vi "tcp_monitor_read_a_frame.vi"(7 "Save":bool, 8 "error in (no error)":errorcluster, 11 "TCP Network Connection in":refnum<k5>) -> (0 "error out":errorcluster, 2 "DataString":string, 3 "TCP Network Connection out":refnum<k5>)   [LabVIEW 2022 SP3]
uses:
  Global 1.vi
panel:
  out "error out 2":errorcluster
  out "length string":string
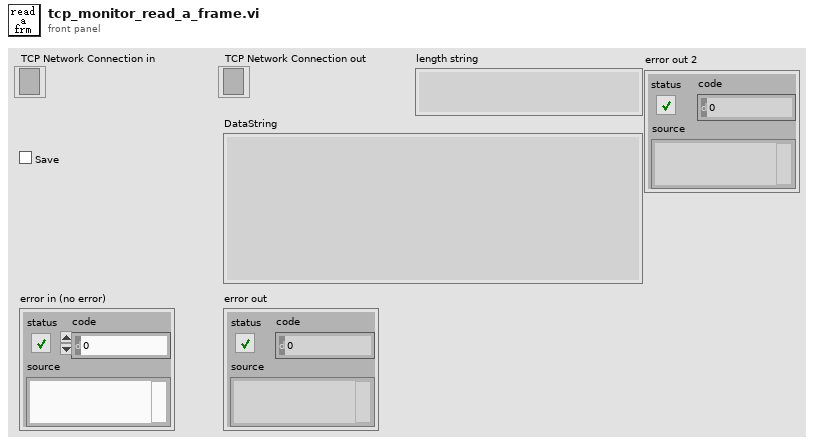
[diagram p1: front panel]
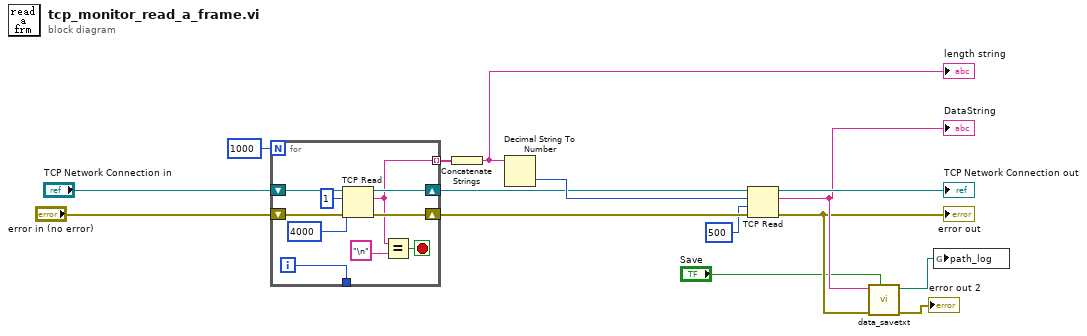
[diagram p0: block diagram]
diagram:
  n1 = for {
    N: 1000 -> [_]
    shift-right: [w24] -> w9
    shift-left: "TCP Network Connection in" -> [w25]
    shift-right: [w22] -> w11
    shift-left: "error in (no error)" -> [w23]
    tunnel: [w18] -> w13 mode=indexing
    tunnel: [w16] -> _
    i -> [w16]
    stop <- w19 stop-if-true
    n2 = TCP Read(connection ID=w25, bytes to read=1, error in (no error)=w23, 9:4000 ("timeout ms (25000)")) -> (connection ID out=w24:refnum<k5>, data out=w18:string, error out=w22:errorcluster)  [unwired: 1 in]
    n3 = Equal?(x=w18, y="\n") -> (x = y?=w19:bool)
  }
  n4 = Concatenate Strings(w13) -> (w15:string)
  "length string" <- w15
  n5 = Decimal String To Number(string=w15) -> (number=w14:i32)  [unwired: 2 in, 1 out]
  n6 = TCP Read(connection ID=w9, bytes to read=w14, error in (no error)=w11, 9:500 ("timeout ms (25000)")) -> (connection ID out=→"TCP Network Connection out":refnum<k5>, data out=w5:string, error out=w4:errorcluster)  [unwired: 1 in]
  "error out" <- w4
  "DataString" <- w5
  n7 = call "data_savetxt.vi"("Save"="Save", "error in (no error)"=w4, "ParasOutput"=w5) -> ("error out"=→"error out 2":errorcluster, "path_out"=w1:path)  [unwired: 7 in]
  n8 = global write "Global 1.vi" "path_log"(w1) -> ()
